vi "Read message.vi"(8 "error in (no error)":errorcluster, 10 "Message type":T1="Control", 11 "Control-Client in":refnum<class "Control-Client.lvclass">) -> (0 "error out":errorcluster, 2 "Message.lvclass":refnum<class "Message.lvclass">, 3 "Control-Client out":refnum<class "Control-Client.lvclass">)   [LabVIEW 2015]
uses:
  Control-Client.lvclass
  Message/Message.lvclass
  dependecies/ControlsVIs/Clusters-def/Message types.ctl
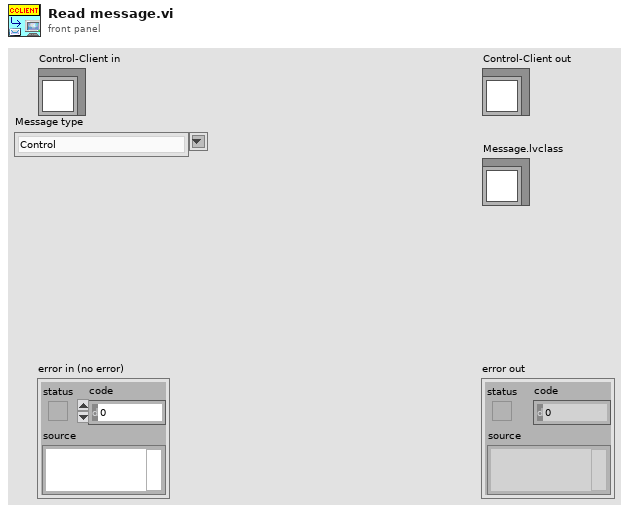
[diagram p1: front panel]
types:
  T1 = typedef "Message types.ctl" = string
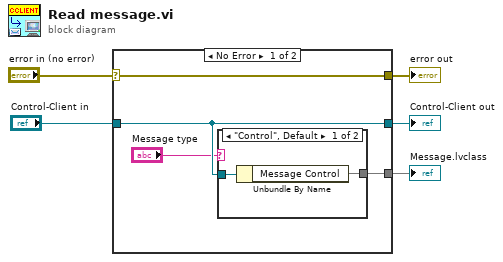
[diagram p0: block diagram]
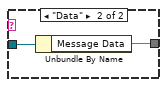
[diagram p2: hidden frame]
diagram:
  n1 = case shown="No Error" "error in (no error)" {
    selector: "error in (no error)" -> [w9 w14]
    tunnel: [w9 w14] -> w4
    tunnel: [w8 w15] -> w2
    tunnel: "Control-Client in" -> [w8 w15]
    tunnel: [w7 _] -> w1
    frame No Error {
      n2 = case shown="\"Control\", Default" "Message type" {
        tunnel: w8 -> [w11 w13]
        tunnel: [w10 w12] -> w7
        frame "Control", Default {
          n3 = Unbundle By Name(w11) -> ("Message Control"=w10)
        }
        frame "Data" {
          n4 = Unbundle By Name(w13) -> ("Message Data"=w12)
        }
      }
    }
    frame Error {
    }
  }
  "error out" <- w4
  "Control-Client out" <- w2
  "Message.lvclass" <- w1
